vi "Kateter_lasare.vi"() -> ()   [LabVIEW 2024]
uses:
  <vilib>/Native 3D Graph/xcontrol/3DPC_SurfacePlot.xctl
  <vilib>/Native 3D Graph/classes/Base Datatype.lvclass
panel:
  out "Vinkel 2":dbl format="%#.0p"
  out "Vinkel":dbl format="%#.0p"
  out "Böjning":dbl format="%#.0f"
  out "3D Kateterspets":refnum<class "Base Datatype.lvclass">[](xcontrol) caption="3D Graph"
  out "Vinkel":picture
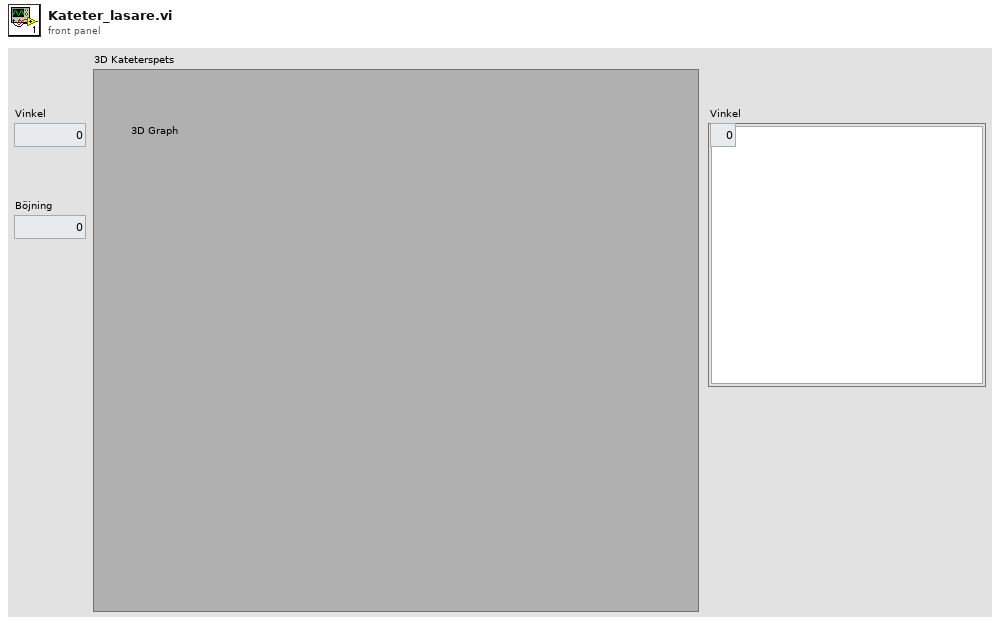
[diagram p1: front panel]
types:
  T1 = cluster{"maximum":dbl, "minimum":dbl, "clip to min":bool, "log?(F)":bool, "grid color":u32, "plot color":u32, "fmt and prec":cluster{"format":enum8{"Decimal", "Scientific", "Engineering", "Binary", "Octal", "Hex"}, "precision":u8}, "visible section":u16}
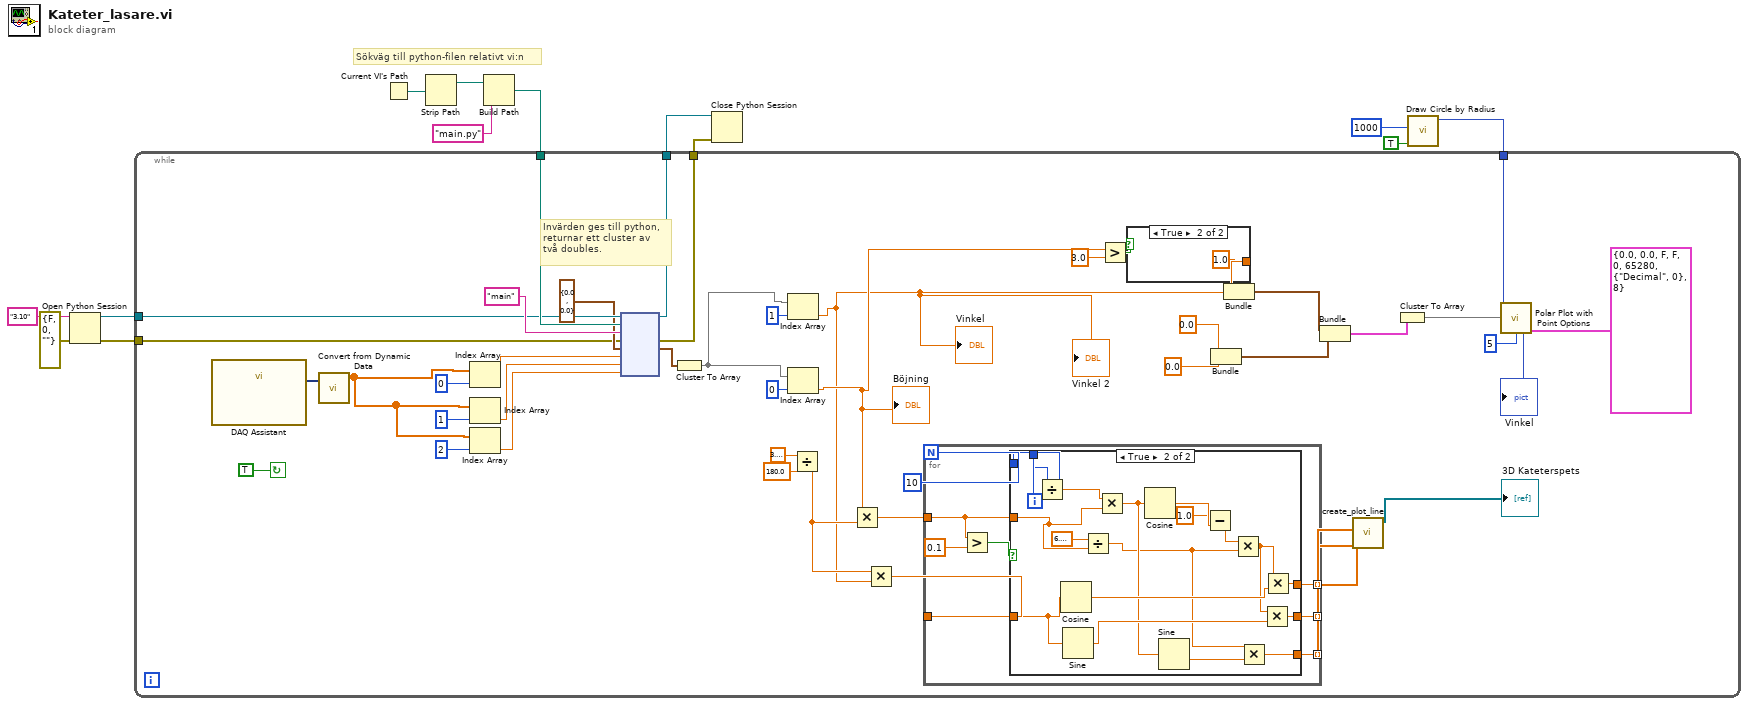
[diagram p0: block diagram]
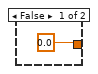
[diagram p2: hidden frame]
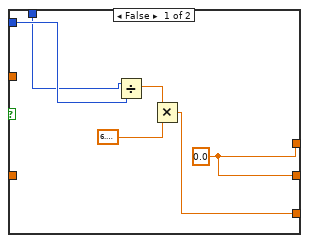
[diagram p3: hidden frame]
diagram:
  # "Sökväg till python-filen relativt vi:n"
  n1 = Open Python Session(python version="3.10" ("Python version"), 3:errorcluster {"status"=FALSE, "code"=0, "source"=""} ("error in (no error)")) -> (session out=w4:refnum<k35>, error out=w3:errorcluster)  [unwired: 1 in]
  n2 = Current VI's Path() -> (path=w9:path)
  n3 = Strip Path(path=w9) -> (stripped path=w10:path)  [unwired: 1 out]
  n4 = Build Path(base path=w10, name or relative path="main.py") -> (appended path=w7:path)
  n5 = call <vilib>:"Draw Circle by Radius.vi"("fill?(F)"=TRUE, "radius"=i16 1000) -> ("new picture"=w11:picture)  [unwired: 9 in]
  n6 = while {
    tunnel: w11 -> [w36]
    tunnel: w7 -> [w26]
    tunnel: w4 -> [w25]
    tunnel: w3 -> [w15]
    tunnel: [w24] -> w2
    tunnel: [w23] -> w1
    stop <- TRUE continue-if-true
    # "Invärden ges till python,\nreturnar ett cluster av \ntvå doubles."
    n7 = call "DAQ Assistant"() -> ("data"=w30:dynamicdata)  [unwired: 17 in, 2 out]
    n8 = call "Convert from Dynamic Data"("Dynamic Data Type"=w30) -> ("Array"=w28:dbl[])  [unwired: 3 in]
    n9 = Index Array(array=w28, index=0) -> (element=w34:dbl)
    n10 = Index Array(array=w28, index=1) -> (element=w33:dbl)
    n11 = Index Array(array=w28, index=2) -> (element=w27:dbl)
    n12 = node(w25, w26, "main" ("function name"), w15, cluster{dbl, dbl} {0.0, 0.0}, w34, w33, w27) -> (w24:refnum<k35>, w23:errorcluster, w20:cluster{dbl, dbl})  [unwired: 3 in, 2 out]
    n13 = Cluster To Array(cluster=w20) -> (array=w19:dbl[])
    n14 = Index Array(array=w19, index=1) -> (element=w17:dbl)
    "Vinkel" <- w17
    "Vinkel 2" <- w17
    n15 = Index Array(array=w19, index=0) -> (element=w18:dbl)
    "Böjning" <- w18
    n16 = Divide(x=3.141592653589793, y=180.0) -> (x/y=w51:dbl)
    n17 = Multiply(x=w18, y=w51) -> (x*y=w50:dbl)
    n18 = Multiply(x=w51, y=w17) -> (x*y=w55:dbl)
    n19 = for {
      N: 10 -> [w69]
      tunnel: w55 -> [w67]
      tunnel: [w66] -> w53 mode=indexing
      tunnel: [w65] -> w54 mode=indexing
      tunnel: [w64] -> w52 mode=indexing
      tunnel: w50 -> [w63]
      i -> [w68]
      n20 = Greater?(x=w63, y=0.1) -> (0:w61:bool)
      n21 = case shown="True" w61 {
        tunnel: w69 -> [w74 w93]
        tunnel: w68 -> [w73 w92]
        tunnel: w67 -> [_ w87]
        tunnel: [w75 w81] -> w66
        tunnel: [w75 w80] -> w65
        tunnel: [w71 w79] -> w64
        tunnel: w63 -> [_ w77]
        frame False {
          w75 = 0.0
          n22 = Divide(x=w73, y=w74) -> (x/y=w70:dbl)
          n23 = Multiply(x=6.283185307179586, y=w70) -> (x*y=w71:dbl)
        }
        frame True {
          n24 = Divide(x=w92, y=w93) -> (x/y=w91:dbl)
          n25 = Cosine(x=w87) -> (cos(x)=w86:dbl)
          n26 = Sine(x=w87) -> (sin(x)=w84:dbl)
          n27 = Divide(x=6.283185307179586, y=w77) -> (x/y=w78:dbl)
          n28 = Multiply(x=w91, y=w77) -> (x*y=w83:dbl)
          n29 = Cosine(x=w83) -> (cos(x)=w90:dbl)
          n30 = Sine(x=w83) -> (sin(x)=w82:dbl)
          n31 = Subtract(x=1.0, y=w90) -> (x-y=w88:dbl)
          n32 = Multiply(x=w88, y=w78) -> (x*y=w85:dbl)
          n33 = Multiply(x=w78, y=w82) -> (x*y=w79:dbl)
          n34 = Multiply(x=w85, y=w84) -> (x*y=w80:dbl)
          n35 = Multiply(x=w85, y=w86) -> (x*y=w81:dbl)
        }
      }
    }
    n36 = Greater?(x=w18, y=3.0) -> (0:w37:bool)
    n37 = case shown="True" w37 {
      tunnel: [0.0 1.0] -> w49
      frame False {
      }
      frame True {
      }
    }
    n38 = Bundle(0.0, 0.0) -> (w45:cluster{dbl, dbl})  [unwired: 1 in]
    n39 = Bundle(w49, w17) -> (w46:cluster{dbl, dbl})  [unwired: 1 in]
    n40 = Bundle(w46, w45) -> (w44:cluster{cluster{dbl, dbl}, cluster{dbl, dbl}})  [unwired: 1 in]
    n41 = call <vilib>:"create_plot_line.vi"("z vector"=w52, "y vector"=w53, "x vector"=w54) -> ("plots out"=→"3D Kateterspets":refnum<class "Base Datatype.lvclass">[])  [unwired: 2 in, 6 out]
    n42 = Cluster To Array(cluster=w44) -> (array=w43:cluster{dbl, dbl}[])
    n43 = call <vilib>:"Polar Plot with Point Options.vi"("picture"=w36, "data array [mag, phase (deg)]"=w43, "polar attributes"=T1 {"maximum"=0.0, "minimum"=0.0, "clip to min"=FALSE, "log?(F)"=FALSE, "grid color"=0, "plot color"=65280, "fmt and prec"={"format"=enum."Decimal", "precision"=0}, "visible section"=8}, "Size"=u16 5) -> ("new picture"=→"Vinkel":picture)  [unwired: 11 in]
  }
  n44 = Close Python Session(session in=w2, error in=w1) -> ()  [unwired: 1 out]
